vi "Z-Scan-core.vi"(0 "trigger in":dbl[](array[numeric]), 1 "ti":i32, 3 "signal in":dbl[](array[numeric]), 4 "tf":i32) -> (5 "mean tf/ti":dbl format="%0.2f", 6 "number of samples":i32=1)   [LabVIEW 2014]
doc: "André Romero - 2016\nandretec@ifsc.usp.br"
uses:
  <vilib>/Analysis/baseanly.llb/Mean (DBL).vi
  <vilib>/Analysis/NI_AALBase.lvlib
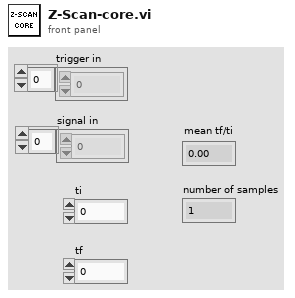
[diagram p1: front panel]
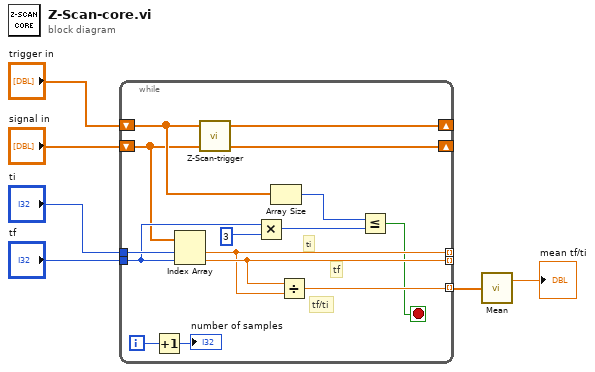
[diagram p0: block diagram]
diagram:
  n1 = while {
    tunnel: "ti" -> [w13]
    tunnel: "tf" -> [w11]
    shift-right: [w7] -> _
    shift-left: "signal in" -> [w9]
    shift-right: [w8] -> _
    shift-left: "trigger in" -> [w10]
    tunnel: [w18] -> _ mode=indexing
    tunnel: [w19] -> _ mode=indexing
    tunnel: [w17] -> w5 mode=indexing
    i -> [w21]
    stop <- w16 stop-if-true
    # "tf"
    # "ti"
    # "tf/ti"
    n2 = Increment(x=w21) -> (x+1=→"number of samples":i32)
    n3 = Index Array(array=w9, index #1=w13, index #2=w11) -> (element #1=w18:dbl, element #2=w19:dbl)
    n4 = call "Z-Scan-trigger.vi"("trigger in"=w10, "signal in"=w9) -> ("trigger out"=w8:dbl[], "signal out"=w7:dbl[])  [unwired: 4 in]
    n5 = Multiply(x=w11, y=3) -> (x*y=w15:i32)
    n6 = Array Size(array=w10) -> (size(s)=w12:i32)
    n7 = Divide(x=w19, y=w18) -> (x/y=w17:dbl)
    n8 = Less Or Equal?(x=w12, y=w15) -> (x <= y?=w16:bool)
  }
  n9 = call-poly <vilib>:"Mean.vi"("X"=w5) -> ("mean"=→"mean tf/ti":dbl)  [unwired: 1 out]
